vi "Man_CtrlEn.vi"(7 "DevState":T1={"Type"=41, "Index"=0, "DeviceOpen"=FALSE, "Ch0Start"=FALSE, "Ch1Start"=FALSE} {"Index" items=["0", "1", "2", "3", "4", "5", "6", "7", "8"]; "Type" items=["USBCANFD-200U"=41, "USBCANFD-100U"=42]}, 8 "error in (no error)":errorcluster caption="错误输入（无错误）", 11 "ManUIref":T2) -> (0 "error out":errorcluster caption="错误输出")   [LabVIEW 2011, in "CAN FD.lvlib"]
uses:
  CAN FD.lvlib
  Typedef/ManUIref.ctl
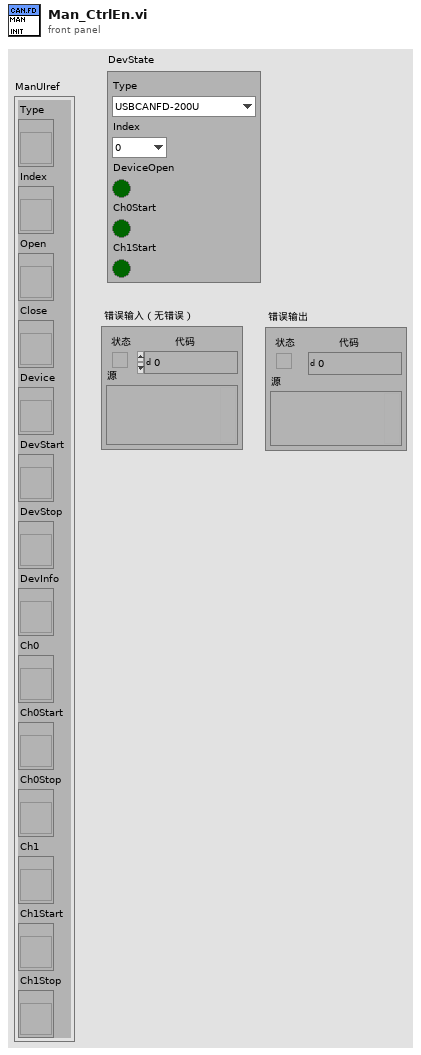
[diagram p1: front panel]
types:
  T1 = cluster{"Type":u32, "Index":u32, "DeviceOpen":bool, "Ch0Start":bool, "Ch1Start":bool}
  T2 = typedef "CAN FD.lvlib/ManUIref.ctl" = cluster{"Type":refnum<vi>, "Index":refnum<vi>, "Open":refnum<vi>, "Close":refnum<vi>, "Device":refnum<vi>, "DevStart":refnum<vi>, "DevStop":refnum<vi>, "DevInfo":refnum<vi>, "Ch0":refnum<vi>, "Ch0Start":refnum<vi>, "Ch0Stop":refnum<vi>, "Ch1":refnum<vi>, "Ch1Start":refnum<vi>, "Ch1Stop":refnum<vi>}
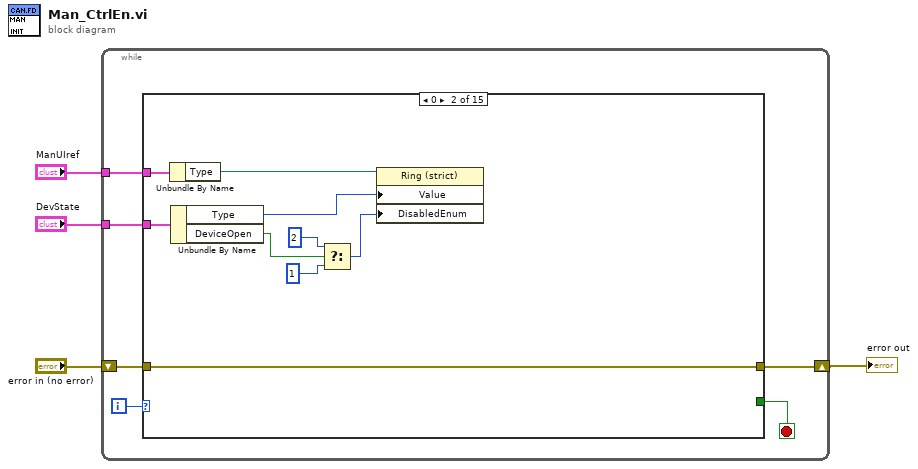
[diagram p0: block diagram]
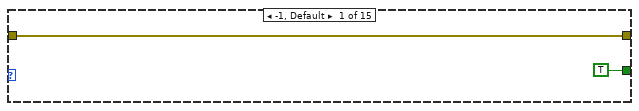
[diagram p2: hidden frame]
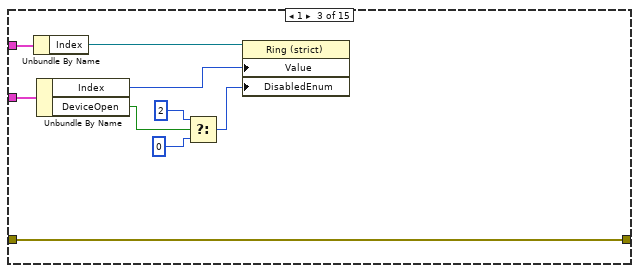
[diagram p3: hidden frame]
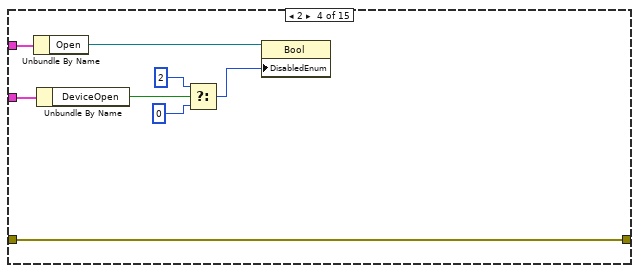
[diagram p4: hidden frame]
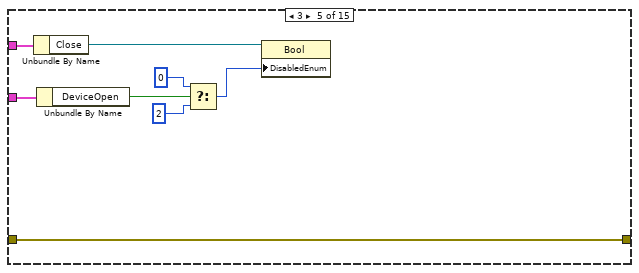
[diagram p5: hidden frame]
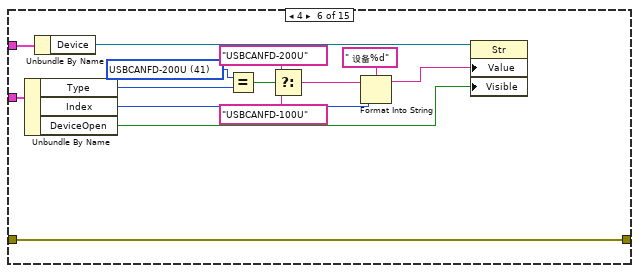
[diagram p6: hidden frame]
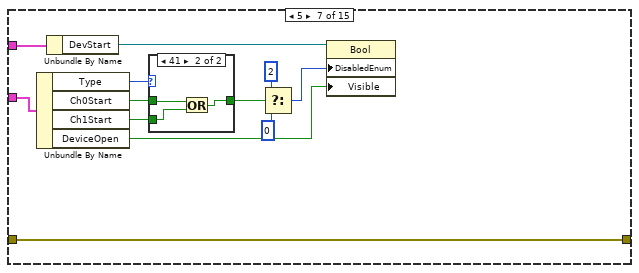
[diagram p7: hidden frame]
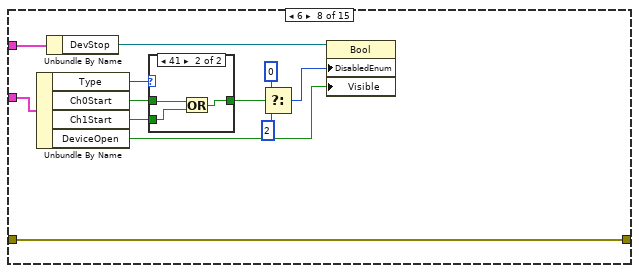
[diagram p9: hidden frame]
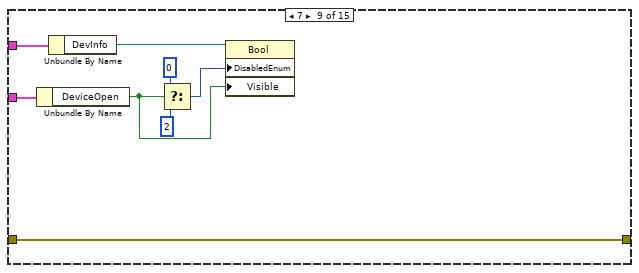
[diagram p11: hidden frame]
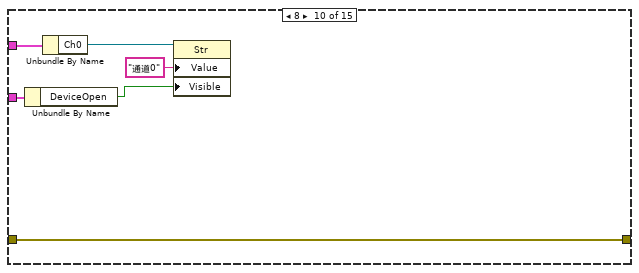
[diagram p12: hidden frame]
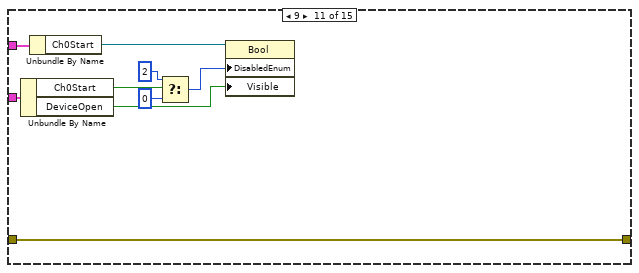
[diagram p13: hidden frame]
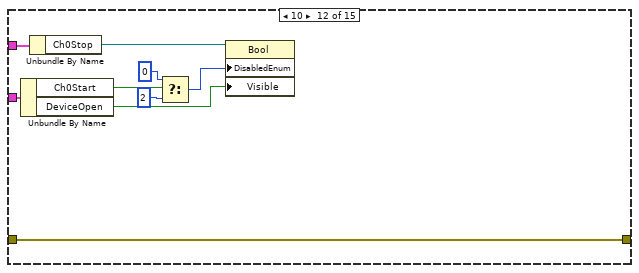
[diagram p14: hidden frame]
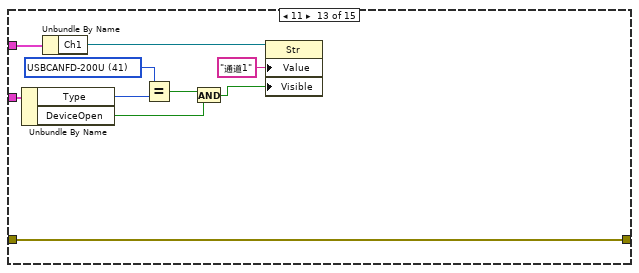
[diagram p15: hidden frame]
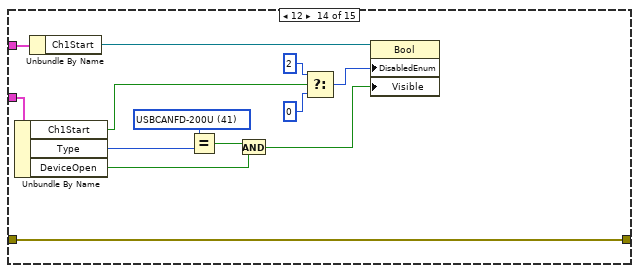
[diagram p16: hidden frame]
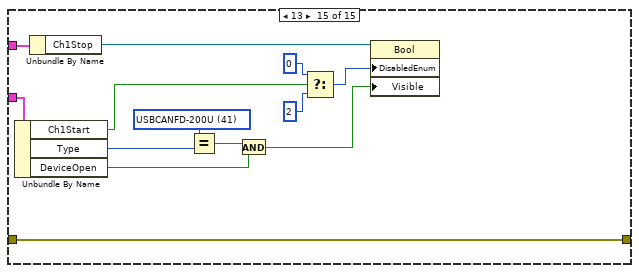
[diagram p17: hidden frame]
diagram:
  n1 = while {
    shift-right: [w8] -> w4
    shift-left: "error in (no error)" -> [w7]
    tunnel: "ManUIref" -> [w6]
    tunnel: "DevState" -> [w5]
    i -> [w10]
    stop <- w9 stop-if-true
    n2 = case shown="0" w10 {
      tunnel: [TRUE _ _ _ _ _ _ _ _ _ _ _ _ _ _] -> w9
      tunnel: [w11 w21 w30 w38 w46 w60 w72 w88 w100 w106 w115 w124 w134 w147 w160] -> w8
      tunnel: w7 -> [w11 w21 w30 w38 w46 w60 w72 w88 w100 w106 w115 w124 w134 w147 w160]
      tunnel: w6 -> [_ w20 w29 w37 w45 w59 w71 w87 w99 w105 w114 w123 w133 w146 w159]
      tunnel: w5 -> [_ w18 w27 w35 w43 w57 w66 w82 w94 w102 w109 w118 w131 w138 w151]
      frame -1, Default {
      }
      frame 0 {
        n3 = Unbundle By Name(w20) -> ("Type"=w19:refnum<vi>)
        n4 = Unbundle By Name(w18) -> ("Type"=w17:u32, "DeviceOpen"=w13:bool)
        n5 = Select(t=2, s=w13, f=1) -> (s? t:f=w14:i32)
        n6 = property class="Ring (strict)"(reference=w19, "Value"=w17, "DisabledEnum"=w14) -> ()  [unwired: 1 in, 2 out]
      }
      frame 1 {
        n7 = Unbundle By Name(w29) -> ("Index"=w28:refnum<vi>)
        n8 = Unbundle By Name(w27) -> ("Index"=w26:u32, "DeviceOpen"=w22:bool)
        n9 = Select(t=2, s=w22, f=0) -> (s? t:f=w23:i32)
        n10 = property class="Ring (strict)"(reference=w28, "Value"=w26, "DisabledEnum"=w23) -> ()  [unwired: 1 in, 2 out]
      }
      frame 2 {
        n11 = Unbundle By Name(w37) -> ("Open"=w36:refnum<vi>)
        n12 = Unbundle By Name(w35) -> ("DeviceOpen"=w31:bool)
        n13 = Select(t=2, s=w31, f=0) -> (s? t:f=w32:i32)
        n14 = property class="Bool"(reference=w36, "DisabledEnum"=w32) -> ()  [unwired: 1 in, 2 out]
      }
      frame 3 {
        n15 = Unbundle By Name(w45) -> ("Close"=w44:refnum<vi>)
        n16 = Unbundle By Name(w43) -> ("DeviceOpen"=w39:bool)
        n17 = Select(t=0, s=w39, f=2) -> (s? t:f=w40:i32)
        n18 = property class="Bool"(reference=w44, "DisabledEnum"=w40) -> ()  [unwired: 1 in, 2 out]
      }
      frame 4 {
        w55 = u32 41 items=["USBCANFD-200U"=41, "USBCANFD-100U"=42] ("Type")
        n19 = Unbundle By Name(w57) -> ("Type"=w56:u32, "Index"=w50:u32, "DeviceOpen"=w47:bool)
        n20 = Unbundle By Name(w59) -> ("Device"=w58:refnum<vi>)
        n21 = Equal?(x=w55, y=w56) -> (x = y?=w54:bool)
        n22 = Select(t="USBCANFD-200U", s=w54, f="USBCANFD-100U") -> (s? t:f=w51:string)
        n23 = Format Into String(format string=" 设备%d" ("格式字符串"), initial string=w51, w50) -> (resulting string=w48:string)  [unwired: 1 in, 1 out]
        n24 = property class="Str"(reference=w58, "Value"=w48, "Visible"=w47) -> ()  [unwired: 1 in, 2 out]
      }
      frame 5 {
        n25 = Unbundle By Name(w66) -> ("Type"=w64:u32, "Ch0Start"=w63:bool, "Ch1Start"=w62:bool, "DeviceOpen"=w65:bool)
        n26 = Unbundle By Name(w71) -> ("DevStart"=w70:refnum<vi>)
        n27 = case shown="41" w64 {
          tunnel: w63 -> [w73 w76]
          tunnel: w62 -> [_ w75]
          tunnel: [w73 w74] -> w61
          frame 0, Default {
          }
          frame 41 {
            n28 = Or(x=w76, y=w75) -> (x .or. y?=w74:bool)
          }
        }
        n29 = Select(t=2, s=w61, f=0) -> (s? t:f=w67:i32)
        n30 = property class="Bool"(reference=w70, "DisabledEnum"=w67, "Visible"=w65) -> ()  [unwired: 1 in, 2 out]
      }
      frame 6 {
        n31 = Unbundle By Name(w82) -> ("Type"=w80:u32, "Ch0Start"=w79:bool, "Ch1Start"=w78:bool, "DeviceOpen"=w81:bool)
        n32 = Unbundle By Name(w87) -> ("DevStop"=w86:refnum<vi>)
        n33 = case shown="41" w80 {
          tunnel: w79 -> [w89 w92]
          tunnel: w78 -> [_ w91]
          tunnel: [w89 w90] -> w77
          frame 0, Default {
          }
          frame 41 {
            n34 = Or(x=w92, y=w91) -> (x .or. y?=w90:bool)
          }
        }
        n35 = Select(t=0, s=w77, f=2) -> (s? t:f=w83:i32)
        n36 = property class="Bool"(reference=w86, "DisabledEnum"=w83, "Visible"=w81) -> ()  [unwired: 1 in, 2 out]
      }
      frame 7 {
        n37 = Unbundle By Name(w94) -> ("DeviceOpen"=w93:bool)
        n38 = Unbundle By Name(w99) -> ("DevInfo"=w98:refnum<vi>)
        n39 = Select(t=0, s=w93, f=2) -> (s? t:f=w95:i32)
        n40 = property class="Bool"(reference=w98, "DisabledEnum"=w95, "Visible"=w93) -> ()  [unwired: 1 in, 2 out]
      }
      frame 8 {
        n41 = Unbundle By Name(w102) -> ("DeviceOpen"=w101:bool)
        n42 = Unbundle By Name(w105) -> ("Ch0"=w104:refnum<vi>)
        n43 = property class="Str"(reference=w104, "Value"="通道0" ("值"), "Visible"=w101) -> ()  [unwired: 1 in, 2 out]
      }
      frame 9 {
        n44 = Unbundle By Name(w109) -> ("Ch0Start"=w108:bool, "DeviceOpen"=w107:bool)
        n45 = Unbundle By Name(w114) -> ("Ch0Start"=w113:refnum<vi>)
        n46 = Select(t=2, s=w108, f=0) -> (s? t:f=w110:i32)
        n47 = property class="Bool"(reference=w113, "DisabledEnum"=w110, "Visible"=w107) -> ()  [unwired: 1 in, 2 out]
      }
      frame 10 {
        n48 = Unbundle By Name(w118) -> ("Ch0Start"=w117:bool, "DeviceOpen"=w116:bool)
        n49 = Unbundle By Name(w123) -> ("Ch0Stop"=w122:refnum<vi>)
        n50 = Select(t=0, s=w117, f=2) -> (s? t:f=w119:i32)
        n51 = property class="Bool"(reference=w122, "DisabledEnum"=w119, "Visible"=w116) -> ()  [unwired: 1 in, 2 out]
      }
      frame 11 {
        w129 = u32 41 items=["USBCANFD-200U"=41, "USBCANFD-100U"=42] ("Type")
        n52 = Unbundle By Name(w131) -> ("Type"=w130:u32, "DeviceOpen"=w125:bool)
        n53 = Unbundle By Name(w133) -> ("Ch1"=w132:refnum<vi>)
        n54 = Equal?(x=w129, y=w130) -> (x = y?=w127:bool)
        n55 = And(x=w127, y=w125) -> (x .and. y?=w126:bool)
        n56 = property class="Str"(reference=w132, "Value"="通道1" ("值"), "Visible"=w126) -> ()  [unwired: 1 in, 2 out]
      }
      frame 12 {
        w140 = u32 41 items=["USBCANFD-200U"=41, "USBCANFD-100U"=42] ("Type")
        n57 = Unbundle By Name(w138) -> ("Ch1Start"=w135:bool, "Type"=w141:u32, "DeviceOpen"=w136:bool)
        n58 = Unbundle By Name(w146) -> ("Ch1Start"=w145:refnum<vi>)
        n59 = Equal?(x=w140, y=w141) -> (x = y?=w139:bool)
        n60 = And(x=w139, y=w136) -> (x .and. y?=w137:bool)
        n61 = Select(t=2, s=w135, f=0) -> (s? t:f=w142:i32)
        n62 = property class="Bool"(reference=w145, "DisabledEnum"=w142, "Visible"=w137) -> ()  [unwired: 1 in, 2 out]
      }
      frame 13 {
        w153 = u32 41 items=["USBCANFD-200U"=41, "USBCANFD-100U"=42] ("Type")
        n63 = Unbundle By Name(w151) -> ("Ch1Start"=w148:bool, "Type"=w154:u32, "DeviceOpen"=w149:bool)
        n64 = Unbundle By Name(w159) -> ("Ch1Stop"=w158:refnum<vi>)
        n65 = Equal?(x=w153, y=w154) -> (x = y?=w152:bool)
        n66 = And(x=w152, y=w149) -> (x .and. y?=w150:bool)
        n67 = Select(t=0, s=w148, f=2) -> (s? t:f=w155:i32)
        n68 = property class="Bool"(reference=w158, "DisabledEnum"=w155, "Visible"=w150) -> ()  [unwired: 1 in, 2 out]
      }
    }
  }
  "error out" <- w4
